vi "SCLN_CheckAuthentication.vi"(0 "Server Name":string, 1 "TCP IN":refnum<k5>) -> (2 "TCP OUT":refnum<k5>, 3 "Client Index":i32, 4 "Authentic":bool, 5 "error out":errorcluster)   [LabVIEW 2015]
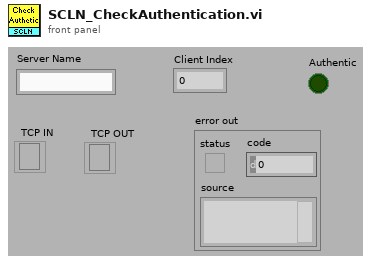
[diagram p1: front panel]
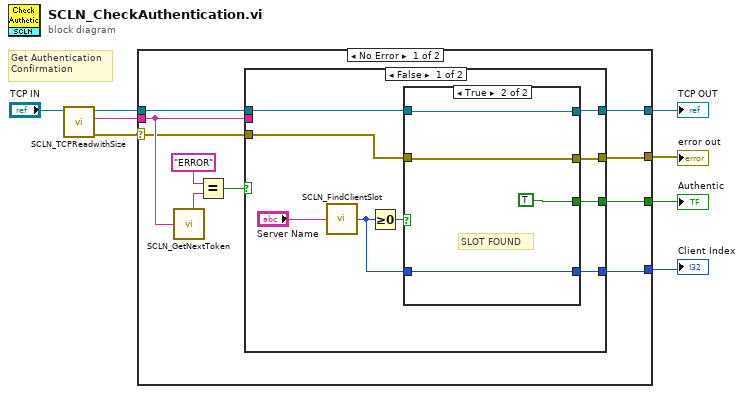
[diagram p0: block diagram]
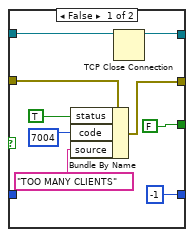
[diagram p2: hidden frame]
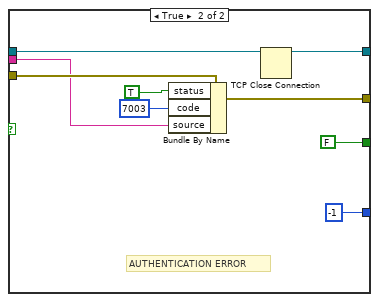
[diagram p3: hidden frame]
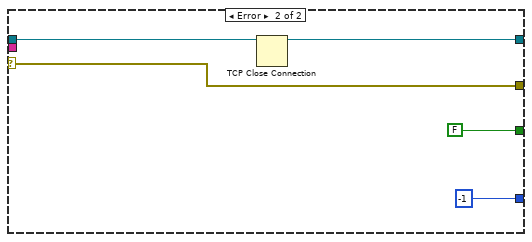
[diagram p4: hidden frame]
diagram:
  # "Get Authentication\nConfirmation"
  n1 = call "SCLN_TCPReadwithSize.vi"("connection ID"="TCP IN") -> ("error out"=w5:errorcluster, "data out"=w6:string, "connection ID out"=w7:refnum<k5>)  [unwired: 8 in]
  n2 = case shown="No Error" w5 {
    selector: w5 -> [w9 w50]
    tunnel: w7 -> [w15 w54]
    tunnel: w6 -> [w14 _]
    tunnel: [w10 w50] -> w4
    tunnel: [w12 FALSE] -> w3
    tunnel: [w11 -1] -> w2
    tunnel: [w13 w51] -> w1
    frame No Error {
      n3 = call "SCLN_GetNextToken.vi"("Input string"=w14) -> ("Token"=w18:string)  [unwired: 4 in, 1 out]
      n4 = Equal?(x="ERROR", y=w18) -> (x = y?=w16:bool)
      n5 = case shown="False" w16 {
        tunnel: w15 -> [w23 w42]
        tunnel: w14 -> [_ w44]
        tunnel: [w19 w41] -> w13
        tunnel: [w21 FALSE] -> w12
        tunnel: [w22 -1] -> w11
        tunnel: w9 -> [w24 w47]
        tunnel: [w20 w43] -> w10
        frame False {
          n6 = call "SCLN_FindClientSlot.vi"("Server Name"="Server Name") -> ("Client Index"=w25:i32)
          n7 = Greater Or Equal To 0?(x=w25) -> (x >= 0?=w26:bool)
          n8 = case shown="True" w26 {
            tunnel: w25 -> [_ w40]
            tunnel: w24 -> [w36 w38]
            tunnel: w23 -> [w32 w37]
            tunnel: [-1 w40] -> w22
            tunnel: [FALSE TRUE] -> w21
            tunnel: [w30 w38] -> w20
            tunnel: [w31 w37] -> w19
            frame False {
              n9 = Bundle By Name(cluster=w36, "status"=TRUE, "code"=7004, "source"="TOO MANY CLIENTS") -> (w30:errorcluster)
              n10 = TCP Close Connection(connection ID=w32) -> (connection ID out=w31:refnum<k5>)  [unwired: 2 in, 1 out]
            }
            frame True {
              # "SLOT FOUND"
            }
          }
        }
        frame True {
          # "AUTHENTICATION ERROR"
          n11 = Bundle By Name(cluster=w47, "status"=TRUE, "code"=7003, "source"=w44) -> (w43:errorcluster)
          n12 = TCP Close Connection(connection ID=w42) -> (connection ID out=w41:refnum<k5>)  [unwired: 2 in, 1 out]
        }
      }
    }
    frame Error {
      n13 = TCP Close Connection(connection ID=w54) -> (connection ID out=w51:refnum<k5>)  [unwired: 2 in, 1 out]
    }
  }
  "Client Index" <- w2
  "Authentic" <- w3
  "TCP OUT" <- w1
  "error out" <- w4
